vi "Move_TRX(LV2013).vi"(7 "DC Motor ID(110)":u32=210, 8 "error in":errorcluster, 9 "Port (LS1)":T1, 10 "Move":cluster{"Pcmd":i32, "Vcmd":i32}={"Pcmd"=1000, "Vcmd"=200}, 11 "KNR in":T2) -> (0 "error out":errorcluster, 3 "KNR out":T2)   [LabVIEW 2013]
uses:
  <userlib>/KNR OS 3.0 LabVIEW Toolkit/Type Definition/KNR3 Reference.ctl
  <userlib>/_FPGA Interface Advanced Tools/FPGA Interface Base/FPGA Interface Base.lvclass
  <userlib>/KNR OS 3.0 LabVIEW Toolkit/Type Definition/Resource.ctl
  <userlib>/KNR OS 3.0 LabVIEW Toolkit/support SubVI/_Controls/Lego Port.ctl
panel:
  out "PWM":i32[](graph)
  out "Waveform Graph":i32[](graph)
  out "TRXDETRXDEGERR":i32
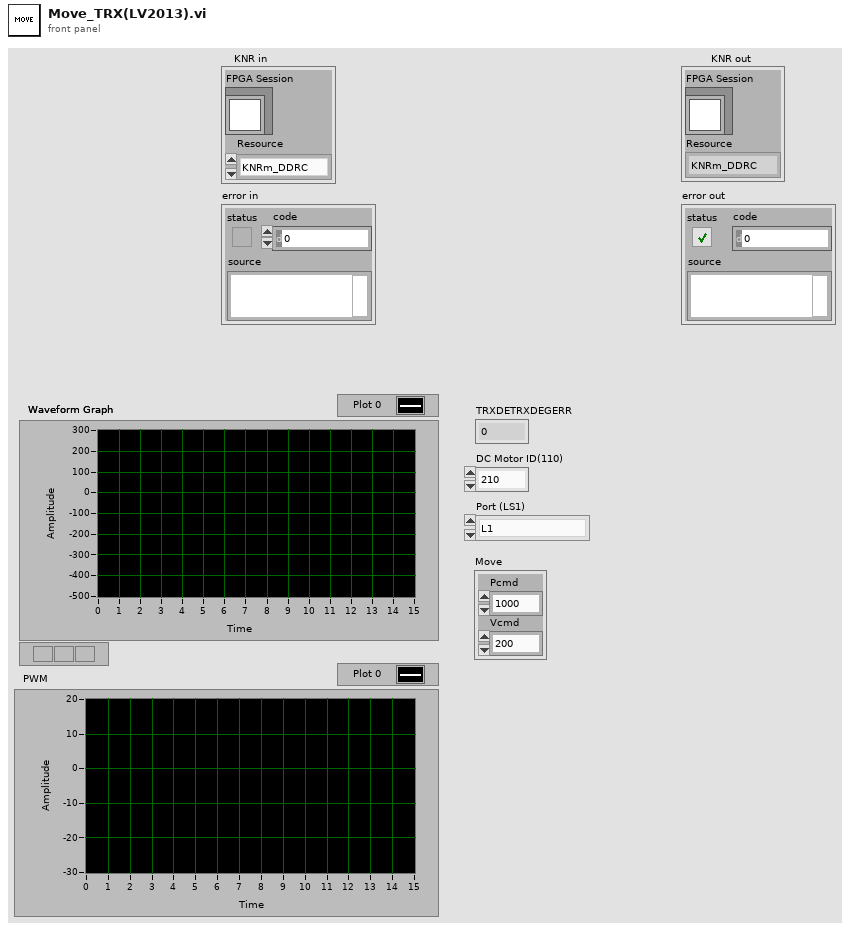
[diagram p1: front panel]
types:
  T1 = typedef "Lego Port.ctl" = enum8{"L1", "LS1", "LS3", "LS4", "LS2"}
  T2 = typedef "KNR3 Reference.ctl" = cluster{"FPGA Session":refnum<class "FPGA Interface Base.lvclass">, "Resource":T3}
  T3 = typedef "Resource.ctl" = enum16{"KNRm_DDRC", "KNRm_DDDD", "KNRm_DDDR", "KNRm_DDDC", "KNR"}
  T4 = cluster{"TS":dbl, "SEC2MSEC":i32, "NXTMINVEL":i32, "NXTMAXVEL":i32, "NXTMAXACC":i32}
  T5 = cluster{"omega":i32, "Kds":i32, "Lhlf":i32, "Ld":i32, "revgain":i32, "ENCX4":i32, "TRXDETRXDEGERR":i32, "dir":cluster{"N[0]":i32, "N[1]":i32, "N[2]":i32, "N[3]":i32}}
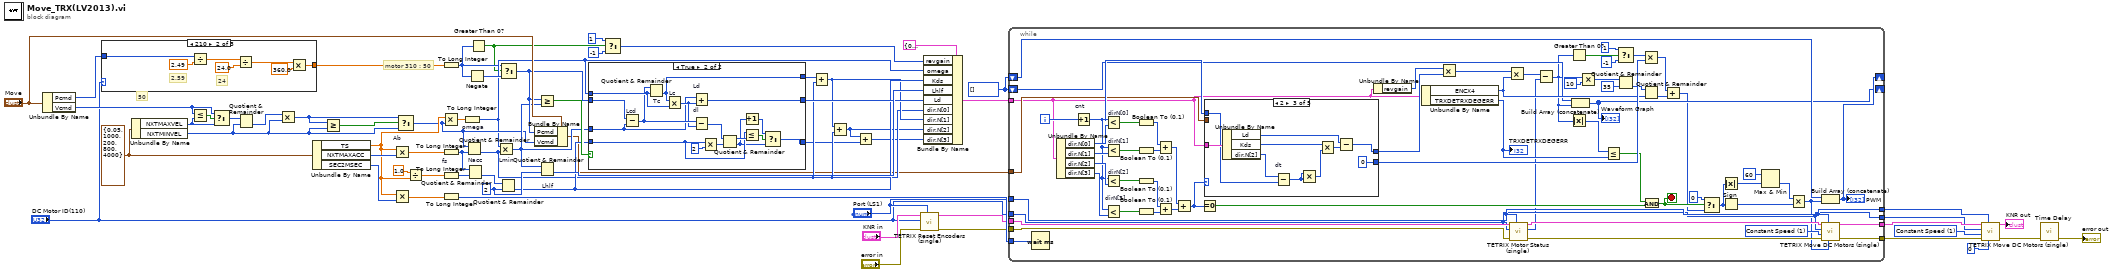
[diagram p0: block diagram]
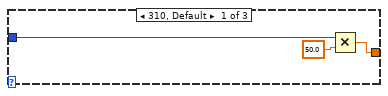
[diagram p2: hidden frame]
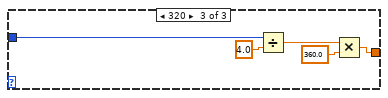
[diagram p3: hidden frame]
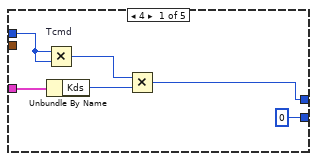
[diagram p4: hidden frame]
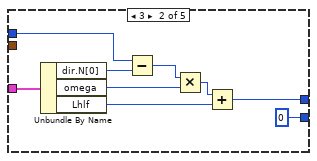
[diagram p5: hidden frame]
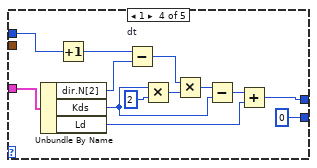
[diagram p6: hidden frame]
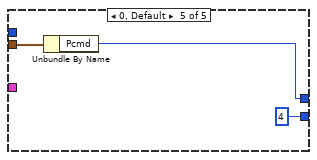
[diagram p7: hidden frame]
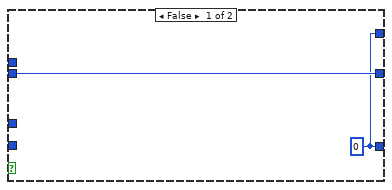
[diagram p8: hidden frame]
diagram:
  w1 = i32[] []
  w8 = u8 1 items=["Constant Power", "Constant Speed"] ("Control Mode (Constant Power)")
  w53 = T4 {"TS"=0.05, "SEC2MSEC"=1000, "NXTMINVEL"=200, "NXTMAXVEL"=800, "NXTMAXACC"=4000} ("input cluster 2")
  w42 = 2 ("y")
  # "50"
  # "motor 310 : 50"
  n1 = Unbundle By Name("Move") -> ("Pcmd"=w4:i32, "Vcmd"=w60:i32)
  n2 = case shown="210" "DC Motor ID(110)" {
    tunnel: w4 -> [w66 w71 w79]
    tunnel: [w65 w68 w77] -> w3
    frame 310, Default {
      n3 = Multiply(x=w66, y=50.0) -> (x*y=w65:dbl)
    }
    frame 210 {
      # "24"
      # "2.59"
      n4 = Divide(x=w71, y=2.49) -> (x/y=w74:dbl)
      n5 = Divide(x=w74, y=24.0) -> (x/y=w69:dbl)
      n6 = Multiply(x=w69, y=360.0) -> (x*y=w68:dbl)
    }
    frame 320 {
      n7 = Divide(x=w79, y=4.0) -> (x/y=w78:dbl)
      n8 = Multiply(x=w78, y=360.0) -> (x*y=w77:dbl)
    }
  }
  n9 = Unbundle By Name(w53) -> ("NXTMAXVEL"=w59:i32, "NXTMINVEL"=w54:i32)
  n10 = Less Or Equal?(x=w60, y=w59) -> (x <= y?=w61:bool)
  n11 = Select(t=w60, s=w61, f=w59) -> (s? t:f=w58:i32)
  n12 = Quotient & Remainder(x=w58, y=w54) -> (floor(x/y)=w57:i32)  [unwired: 1 out]
  n13 = Multiply(x=w57, y=w54) -> (x*y=w55:i32)
  n14 = Unbundle By Name(w53) -> ("TS"=w48:dbl, "NXTMAXACC"=w51:i32, "SEC2MSEC"=w52:i32)
  n15 = Greater Or Equal?(x=w55, y=w54) -> (x >= y?=w56:bool)
  n16 = Multiply "Ab"(x=w48, y=w51) -> (x*y=w46:dbl)
  n17 = Multiply(x=w48, y=w52) -> (x*y=w22:dbl)
  n18 = Select(t=w55, s=w56, f=w54) -> (s? t:f=w38:i32)
  n19 = Divide(x=1.0, y=w48) -> (x/y=w49:dbl)
  n20 = To Long Integer(number=w3) -> (32bit integer=w27:i32)
  n21 = Multiply(x=w48, y=w38) -> (x*y=w47:dbl)
  n22 = To Long Integer(number=w46) -> (32bit integer=w45:i32)
  n23 = To Long Integer "fs"(number=w49) -> (32bit integer=w44:i32)
  n24 = To Long Integer(number=w22) -> (32bit integer=w21:i32)
  n25 = To Long Integer "omega"(number=w47) -> (32bit integer=w37:i32)
  n26 = Quotient & Remainder "Nacc"(x=w38, y=w45) -> (floor(x/y)=w31:i32)  [unwired: 1 out]
  n27 = Quotient & Remainder(x=w45, y=w44) -> (floor(x/y)=w35:i32)  [unwired: 1 out]
  n28 = Negate(x=w27) -> (-x=w64:i32)
  n29 = Greater Than 0?(x=w27) -> (x > 0?=w26:bool)
  n30 = Multiply "Lmin"(x=w37, y=w31) -> (x*y=w39:i32)
  n31 = Quotient & Remainder(x=w35, y=w42) -> (floor(x/y)=w34:i32)  [unwired: 1 out]
  n32 = Select(t=w27, s=w26, f=w64) -> (s? t:f=w40:i32)
  n33 = Bundle By Name(cluster="Move", "Pcmd"=w40, "Vcmd"=w38) -> (w20:cluster{"Pcmd":i32, "Vcmd":i32})
  n34 = Greater Or Equal?(x=w40, y=w39) -> (x >= y?=w43:bool)
  n35 = Quotient & Remainder "Lhlf"(x=w39, y=w42) -> (floor(x/y)=w41:i32)  [unwired: 1 out]
  n36 = case shown="True" w43 {
    tunnel: w40 -> [w81 w97]
    tunnel: w39 -> [_ w92]
    tunnel: w37 -> [_ w96]
    tunnel: [w80 w95] -> w33
    tunnel: [w81 w91] -> w36
    tunnel: w34 -> [_ w86]
    tunnel: [w80 w82] -> w28
    frame False {
      w80 = 0
    }
    frame True {
      n37 = Subtract "Lcd"(x=w97, y=w92) -> (x-y=w94:i32)
      n38 = Quotient & Remainder "Tc"(x=w94, y=w96) -> (floor(x/y)=w95:i32)  [unwired: 1 out]
      n39 = Multiply "Lc"(x=w95, y=w96) -> (x*y=w93:i32)
      n40 = Add "Ld"(x=w92, y=w93) -> (x+y=w91:i32)
      n41 = Subtract "dl"(x=w94, y=w93) -> (x-y=w90:i32)
      n42 = Multiply(x=w86, y=2) -> (x*y=w89:i32)
      n43 = Quotient & Remainder(x=w90, y=w89) -> (x-y*floor(x/y)=w87:i32, floor(x/y)=w83:i32)
      n44 = Increment(x=w83) -> (x+1=w84:i32)
      n45 = Less Or Equal?(x=w86, y=w87) -> (x <= y?=w85:bool)
      n46 = Select(t=w84, s=w85, f=w83) -> (s? t:f=w82:i32)
    }
  }
  n47 = Select(t=1, s=w26, f=-1 ("t")) -> (s? t:f=w24:i32)
  n48 = Add(x=w33, y=w31) -> (x+y=w32:i32)
  n49 = Add(x=w32, y=w31) -> (x+y=w30:i32)
  n50 = Add(x=w30, y=w28) -> (x+y=w29:i32)
  n51 = call <userlib>:"TETRIX Reset Encoders (single).vi"("Port (LS1)"="Port (LS1)", "error in"="error in", "DC Motor ID(110)"="DC Motor ID(110)", "KNR in"="KNR in") -> ("error out"=w15:errorcluster, "KNR out"=w17:T2)  [unwired: 6 in]
  n52 = Bundle By Name(cluster=T5 {"omega"=0, "Kds"=0, "Lhlf"=0, "Ld"=0, "revgain"=0, "ENCX4"=4, "TRXDETRXDEGERR"=24, "dir"={"N[0]"=0, "N[1]"=0, "N[2]"=0, "N[3]"=0}} ("Cluster"), "revgain"=w24, "omega"=w37, "Kds"=w34, "Lhlf"=w41, "Ld"=w36, "dir.N[0]"=w31, "dir.N[1]"=w32, "dir.N[2]"=w30, "dir.N[3]"=w29) -> (w19:T5)
  n53 = while {
    tunnel: w21 -> [w161]
    tunnel: w20 -> [w137]
    tunnel: w19 -> [w129]
    tunnel: [w123] -> w13
    tunnel: w17 -> [w124]
    tunnel: "Port (LS1)" -> [w113]
    tunnel: "DC Motor ID(110)" -> [w112]
    tunnel: w15 -> [w118]
    tunnel: [w115] -> w12
    tunnel: [w113] -> w10
    tunnel: [w112] -> w9
    shift-right: [w107] -> _
    shift-left: w1 -> [w111]
    shift-right: [w108] -> _
    shift-left: w1 -> [w109]
    i -> [w152]
    stop <- w116 stop-if-true
    w120 = u8 1 items=["Constant Power", "Constant Speed"] ("Control Mode (Constant Power)")
    n54 = Wait (ms)(milliseconds to wait=w161) -> ()  [unwired: 1 out]
    n55 = Unbundle By Name(w129) -> ("dir.N[0]"=w151:i32, "dir.N[1]"=w150:i32, "dir.N[2]"=w149:i32, "dir.N[3]"=w148:i32)
    n56 = Increment "cnt"(x=w152) -> (x+1=w145:i32)
    n57 = Less? "dirN[0]"(x=w145, y=w151) -> (x < y?=w157:bool)
    n58 = Less? "dirN[1]"(x=w145, y=w150) -> (x < y?=w154:bool)
    n59 = Less? "dirN[2]"(x=w145, y=w149) -> (x < y?=w155:bool)
    n60 = Less? "dirN[3]"(x=w145, y=w148) -> (x < y?=w156:bool)
    n61 = Boolean To (0,1)(Boolean=w157) -> (0, 1=w153:i16)
    n62 = Boolean To (0,1)(Boolean=w154) -> (0, 1=w158:i16)
    n63 = Boolean To (0,1)(Boolean=w155) -> (0, 1=w159:i16)
    n64 = Boolean To (0,1)(Boolean=w156) -> (0, 1=w160:i16)
    n65 = Add(x=w153, y=w158) -> (x+y=w147:i16)
    n66 = Add(x=w159, y=w160) -> (x+y=w146:i16)
    n67 = Add(x=w147, y=w146) -> (x+y=w139:i16)
    n68 = Equal To 0?(x=w139) -> (x = 0?=w138:bool)
    n69 = case shown="2" w139 {
      tunnel: [w165 w170 w186 w189 w201] -> w144
      tunnel: w145 -> [w167 w176 w181 w199 _]
      tunnel: w129 -> [w166 w175 w185 w196 _]
      tunnel: w137 -> [_ _ _ _ w202]
      tunnel: [0 ("L_Friction") 0 ("L_Friction") 0 ("L_Friction") 0 ("L_Friction") 4 ("L_Friction")] -> w132
      frame 4 {
        n70 = Multiply "Tcmd"(x=w167, y=w167) -> (x*y=w164:i32)
        n71 = Unbundle By Name(w166) -> ("Kds"=w163:i32)
        n72 = Multiply(x=w164, y=w163) -> (x*y=w165:i32)
      }
      frame 3 {
        n73 = Unbundle By Name(w175) -> ("dir.N[0]"=w168:i32, "omega"=w173:i32, "Lhlf"=w172:i32)
        n74 = Subtract(x=w176, y=w168) -> (x-y=w174:i32)
        n75 = Multiply(x=w174, y=w173) -> (x*y=w171:i32)
        n76 = Add(x=w171, y=w172) -> (x+y=w170:i32)
      }
      frame 2 {
        n77 = Unbundle By Name(w185) -> ("Ld"=w184:i32, "Kds"=w178:i32, "dir.N[2]"=w182:i32)
        n78 = Subtract "dt"(x=w182, y=w181) -> (x-y=w180:i32)
        n79 = Multiply(x=w180, y=w180) -> (x*y=w179:i32)
        n80 = Multiply(x=w178, y=w179) -> (x*y=w177:i32)
        n81 = Subtract(x=w184, y=w177) -> (x-y=w186:i32)
      }
      frame 1 {
        n82 = Unbundle By Name(w196) -> ("dir.N[2]"=w190:i32, "Kds"=w194:i32, "Ld"=w193:i32)
        n83 = Increment(x=w199) -> (x+1=w198:i32)
        n84 = Subtract "dt"(x=w198, y=w190) -> (x-y=w197:i32)
        n85 = Multiply(x=w194, y=2) -> (x*y=w195:i32)
        n86 = Multiply(x=w197, y=w195) -> (x*y=w188:i32)
        n87 = Subtract(x=w188, y=w194) -> (x-y=w187:i32)
        n88 = Add(x=w187, y=w193) -> (x+y=w189:i32)
      }
      frame 0, Default {
        n89 = Unbundle By Name(w202) -> ("Pcmd"=w201:i32)
      }
    }
    n90 = Unbundle By Name(w129) -> ("revgain"=w143:i32)
    n91 = Unbundle By Name(w129) -> ("ENCX4"=w125:i32, "TRXDETRXDEGERR"=w128:i32)
    "TRXDETRXDEGERR" <- w128
    n92 = Multiply(x=w143, y=w144) -> (x*y=w131:i32)
    n93 = Multiply(x=w131, y=w125) -> (x*y=w130:i32)
    n94 = call <userlib>:"TETRIX Motor Status (single).vi"("Port (LS1)"=w113, "error in"=w118, "DC Motor ID(110)"=w112, "KNR in"=w124) -> ("error out"=w117:errorcluster, "Absolute Motor Position"=w99:i32, "KNR out"=w122:T2)  [unwired: 4 in, 1 out]
    n95 = Subtract(x=w130, y=w99) -> (x-y=w110:i32)
    n96 = Greater Than 0?(x=w110) -> (x > 0?=w136:bool)
    n97 = Absolute Value(x=w110) -> (abs(x)=w140:i32)
    n98 = Build Array (concatenate)(w111, w110) -> (w107:i32[])
    "Waveform Graph" <- w107
    n99 = Multiply(x=w110, y=10) -> (x*y=w141:i32)
    n100 = Less Or Equal?(x=w140, y=w128) -> (x <= y?=w121:bool)
    n101 = Select(t=1, s=w136, f=-1 ("t")) -> (s? t:f=w133:i32)
    n102 = Quotient & Remainder(x=w141, y=35) -> (floor(x/y)=w127:i32)  [unwired: 1 out]
    n103 = Multiply(x=w133, y=w132) -> (x*y=w106:i32)
    n104 = Quotient & Remainder(x=w127, y=w125) -> (floor(x/y)=w126:i32)  [unwired: 1 out]
    n105 = And(x=w121, y=w138) -> (x .and. y?=w116:bool)
    n106 = Add(x=w106, y=w126) -> (x+y=w98:i32)
    n107 = Select(t=0, s=w116, f=w98) -> (s? t:f=w103:i32)
    n108 = Absolute Value(x=w103) -> (abs(x)=w104:i32)
    n109 = Sign(1:w103) -> (0:w101:i32)
    n110 = Max & Min(x=60, y=w104) -> (min(x,y)=w102:i32)  [unwired: 1 out]
    n111 = Multiply(x=w102, y=w101) -> (x*y=w100:i32)
    n112 = Build Array (concatenate)(w109, w100) -> (w108:i32[])
    "PWM" <- w108
    n113 = call <userlib>:"TETRIX Move DC Motors (single).vi"("Power/Speed(0)"=w100, "Port (LS1)"=w113, "error in"=w117, "Control Mode (Constant Power)"=w120, "DC Motor ID(110)"=w112, "KNR in"=w122) -> ("error out"=w115:errorcluster, "KNR out"=w123:T2)  [unwired: 4 in]
  }
  n114 = call <userlib>:"TETRIX Move DC Motors (single).vi"("Power/Speed(0)"=i8 0, "Port (LS1)"=w10, "error in"=w12, "Control Mode (Constant Power)"=w8, "DC Motor ID(110)"=w9, "KNR in"=w13) -> ("error out"=w6:errorcluster, "KNR out"=→"KNR out":T2)  [unwired: 4 in]
  n115 = call "Time Delay"("error in (no error)"=w6) -> ("error out"=→"error out":errorcluster)  [unwired: 10 in]
